vi "FTW-Collection-KeyEncode.vi"(1 "Key":string) -> (0 "Encoded Key":string)   [LabVIEW 2012]
uses:
  JSON/FTW-JSON-Escape.vi
panel:
  # "Inputs"
  # "Outputs"
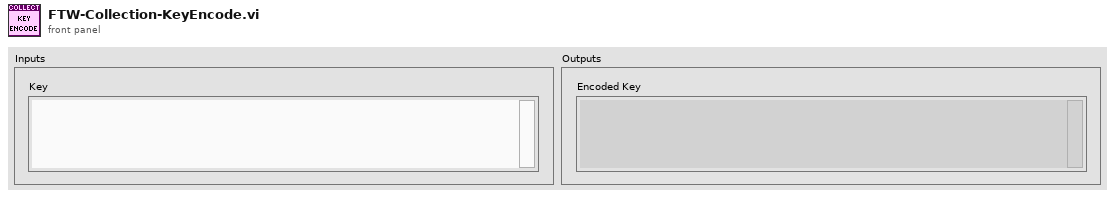
[diagram p1: front panel]
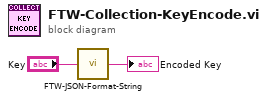
[diagram p0: block diagram]
diagram:
  n1 = call "FTW-JSON-Format-String.vi"("LabVIEW String"="Key") -> ("JSON String"=→"Encoded Key":string)
